vi "Define Units.vi"(8 "error in":errorcluster, 11 "AI Vrms channel in":refnum<class "AI Vrms Channel.lvclass">) -> (0 "error out":errorcluster, 3 "AI Vrms channel out":refnum<class "AI Vrms Channel.lvclass">)   [LabVIEW 2020, in "Scan Engine Scripting.lvlib" / "AI Vrms Channel.lvclass"]
uses:
  AI Vrms Channel.lvclass
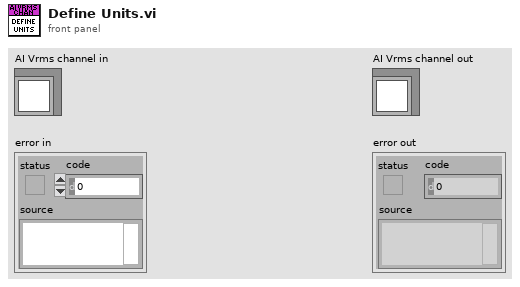
[diagram p1: front panel]
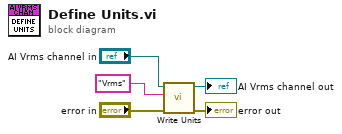
[diagram p0: block diagram]
diagram:
  n1 = call-dynamic "Write Units.vi"("error in"="error in", "units"="Vrms", "channel in"="AI Vrms channel in") -> ("error out"=→"error out":errorcluster, "channel out"=→"AI Vrms channel out":refnum<class "AI Vrms Channel.lvclass">)  [unwired: 7 in]
